vi "Read Fail Meas Points.vi"(7 "Channel (1)":i32=1, 8 "error in (no error)":errorcluster, 11 "VISA resource name":refnum<visa-resource-name>) -> (0 "error out":errorcluster, 1 "Number of Failed Points":i32, 2 "Data":dbl[](array[numeric]), 3 "VISA resource name out":refnum<visa-resource-name>)   [LabVIEW 2011, in "Agilent ENA Series.lvlib"]
doc: "For the active trace of selected channel, reads out the number of the measurement points and stimulus values (frequency, power level or time) at all the measurement point that failed the limit test."
uses:
  Agilent ENA Series.lvlib
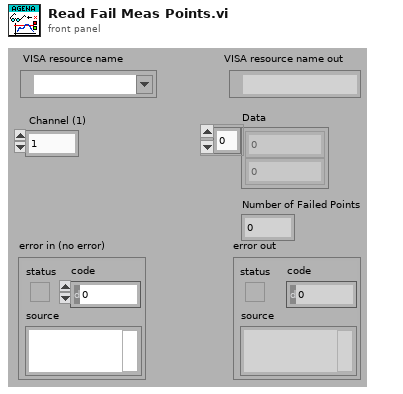
[diagram p1: front panel]
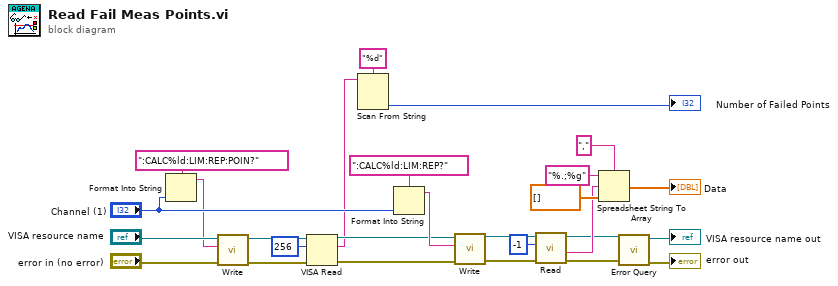
[diagram p0: block diagram]
diagram:
  n1 = Format Into String(format string=":CALC%ld:LIM:REP:POIN?", "Channel (1)") -> (resulting string=w3:string)  [unwired: 2 in, 1 out]
  n2 = call "Write.vi"("error in (no error)"="error in (no error)", "String ()"=w3, "VISA resource name"="VISA resource name") -> ("error out"=w12:errorcluster, "VISA resource name out"=w13:refnum<visa-resource-name>)  [unwired: 6 in, 1 out]
  n3 = VISA Read(VISA resource name=w13, byte count=u32 256, error in (no error)=w12) -> (VISA resource name out=w7:refnum<visa-resource-name>, read buffer=w1:string, error out=w8:errorcluster)  [unwired: 1 out]
  n4 = Scan From String(format string="%d", input string=w1) -> (output 1=→"Number of Failed Points":i32)  [unwired: 3 in, 3 out]
  n5 = Format Into String(format string=":CALC%ld:LIM:REP?", "Channel (1)") -> (resulting string=w26:string)  [unwired: 2 in, 1 out]
  n6 = call "Write.vi"("error in (no error)"=w8, "String ()"=w26, "VISA resource name"=w7) -> ("error out"=w21:errorcluster, "VISA resource name out"=w22:refnum<visa-resource-name>)  [unwired: 6 in, 1 out]
  n7 = call "Read.vi"("error in (no error)"=w21, "Number Of Bytes"=-1, "VISA resource name"=w22) -> ("error out"=w16:errorcluster, "String"=w20:string, "VISA resource name out"=w17:refnum<visa-resource-name>)  [unwired: 5 in, 1 out]
  n8 = Spreadsheet String To Array(delimiter (Tab)=",", format string="%.;%g", spreadsheet string=w20, array type (2D Dbl)=dbl[] []) -> (array=→"Data":dbl[])
  n9 = call "Error Query.vi"("error in (no error)"=w16, "VISA resource name"=w17) -> ("error out"=→"error out":errorcluster, "VISA resource name out"=→"VISA resource name out":refnum<visa-resource-name>)  [unwired: 6 in, 2 out]
